vi "Launch Data Type Selector.vi"(8 "error in (no error)":errorcluster, 9 "Mods":cluster{"Double Click":bool, "Menu Key":bool}, 10 "Coords":T1, 11 "DataGrid Config Dialog in":refnum<class "DataGrid Config Dialog.lvclass">) -> (0 "error out":errorcluster, 3 "DataGrid Config Dialog out":refnum<class "DataGrid Config Dialog.lvclass">)   [LabVIEW 2018, in "DataGrid Config Dialog.lvclass"]
uses:
  DataGrid Config Dialog.lvclass
  <vilib>/Utility/miscctls.llb/LVPoint32TypeDef.ctl
  DataGrid Config Dialog.lvclass/DataGrid Config Dialog.ctl
  Data Type Selector/Data Type Selector.lvclass
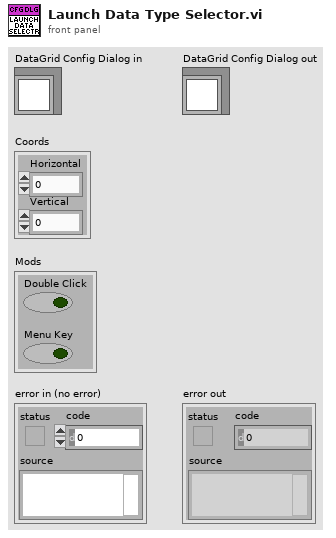
[diagram p1: front panel]
types:
  T1 = typedef "LVPoint32TypeDef.ctl" = cluster{"Horizontal":i32, "Vertical":i32}
  T2 = typedef "LVRowAndColumnTypeDef.ctl" = cluster{"Row":i32, "Column":i32}
  T3 = typedef "LVPositionTypeDef.ctl" = cluster{"Left":i32, "Top":i32}
  T4 = typedef "LVBoundsTypeDef.ctl" = cluster{"Width":u32, "Height":u32}
  T5 = typedef "LVPointTypeDef.ctl" = cluster{"Horizontal":i16, "Vertical":i16}
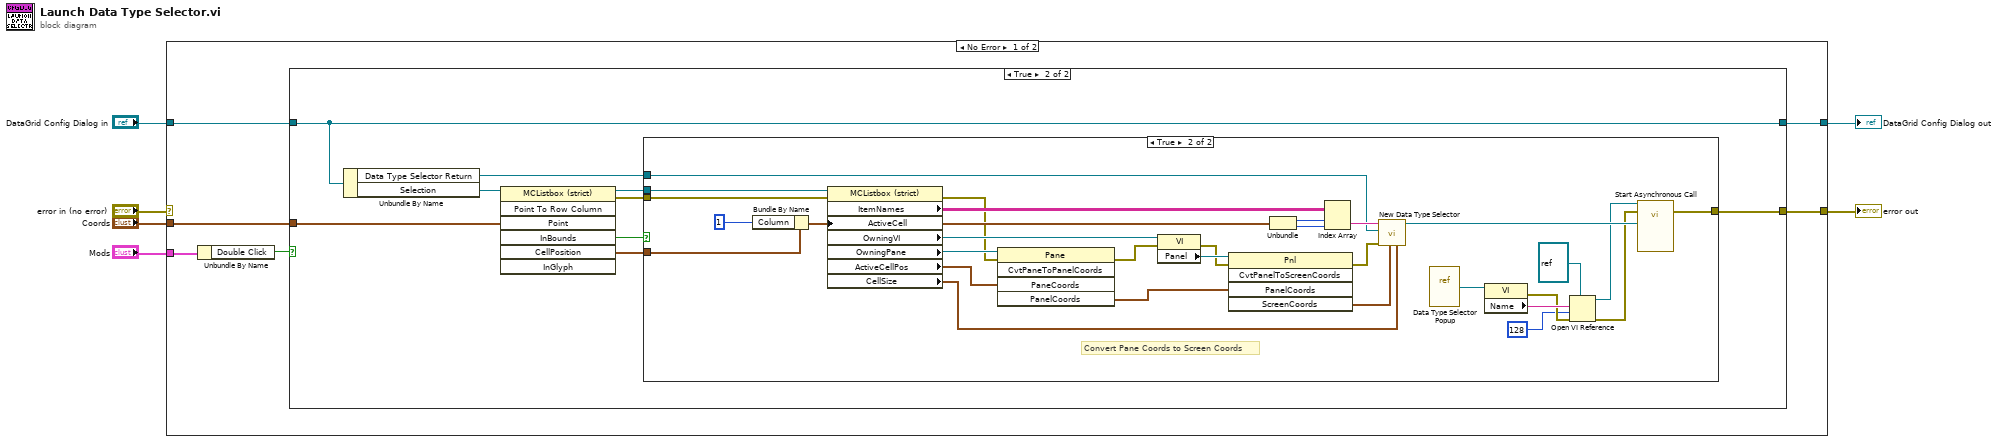
[diagram p0: block diagram]
diagram:
  n1 = case shown="No Error" "error in (no error)" {
    selector: "error in (no error)" -> [_ w55]
    tunnel: [w10 w55] -> w5
    tunnel: [w9 w54] -> w4
    tunnel: "DataGrid Config Dialog in" -> [w8 w54]
    tunnel: "Mods" -> [w12 _]
    tunnel: "Coords" -> [w7 _]
    frame No Error {
      n2 = Unbundle By Name(w12) -> ("Double Click"=w11:bool)
      n3 = case shown="True" w11 {
        tunnel: [_ w17] -> w10
        tunnel: [w13 w21] -> w9
        tunnel: w8 -> [w13 w21]
        tunnel: w7 -> [_ w16]
        frame False {
        }
        frame True {
          n4 = Unbundle By Name(w21) -> ("Data Type Selector Return"=w18:refnum<user-event>, "Selection"=w22:refnum<vi>)
          n5 = invoke class="MCListbox (strict)" method="Point To Row Column"(reference=w22, "Point"=w16) -> (reference out=w20:refnum<vi>, error out=w19:errorcluster, "InBounds"=w14:bool, "CellPosition"=w15:T2)  [unwired: 5 in, 3 out]
          n6 = case shown="True" w14 {
            tunnel: w20 -> [_ w50]
            tunnel: w19 -> [w23 w49]
            tunnel: w18 -> [_ w45]
            tunnel: [w23 w24] -> w17
            tunnel: w15 -> [_ w32]
            frame False {
            }
            frame True {
              # "Convert Pane Coords to Screen Coords"
              n7 = Bundle By Name(cluster=w32, "Column"=1) -> (w48:T2)
              n8 = property class="MCListbox (strict)"(reference=w50, error in=w49, "ActiveCell"=w48) -> (error out=w34:errorcluster, "ItemNames"=w53:string[][], "OwningVI"=w41:refnum<vi>, "OwningPane"=w43:refnum<vi>, "ActiveCellPos"=w42:T3, "CellSize"=w35:T4)  [unwired: 1 out]
              n9 = invoke class="Pane" method="CvtPaneToPanelCoords"(reference=w43, error in=w34, "PaneCoords"=w42) -> (error out=w40:errorcluster, "PanelCoords"=w38:T5)  [unwired: 2 in, 3 out]
              n10 = property class="VI"(reference=w41, error in=w40) -> (error out=w37:errorcluster, "Panel"=w39:refnum<vi>)  [unwired: 1 out]
              n11 = invoke class="Pnl" method="CvtPanelToScreenCoords"(reference=w39, error in=w37, "PanelCoords"=w38) -> (error out=w33:errorcluster, "ScreenCoords"=w36:T5)  [unwired: 2 in, 3 out]
              n12 = Unbundle(w48) -> ("Row"=w47:i32, "Column"=w46:i32)
              n13 = Index Array(array=w53, index (row)=w47, index (col)=w46) -> (element=w52:string)
              n14 = call "New Data Type Selector.vi"("Size"=w35, "Position"=w36, "error in (no error)"=w33, "Data Type Selector Return"=w45, "Data Type in"=w52) -> ("Data Type Selector out"=w44:refnum<class "Data Type Selector.lvclass">)  [unwired: 5 in, 1 out]
              n15 = vi-ref "Data Type Selector Popup.vi"() -> (w31:refnum<vi>)
              n16 = property class="VI"(reference=w31) -> (error out=w29:errorcluster, "Name"=w30:string)  [unwired: 1 in, 1 out]
              n17 = Open VI Reference(type specifier VI Refnum (for type only)=refnum<vi> refnum, vi path=w30, options=128, error in (no error)=w29) -> (vi reference=w26:refnum<vi>, error out=w25:errorcluster)  [unwired: 2 in]
              n18 = call-by-ref "Start Asynchronous Call"(reference=w26, error in=w25, "Data Type Selector in"=w44) -> (error out=w24:errorcluster)  [unwired: 11 in, 1 out]
            }
          }
        }
      }
    }
    frame Error {
    }
  }
  "error out" <- w5
  "DataGrid Config Dialog out" <- w4
